vi "Set Controller Configuration.vi"(8 "error in (no error)":errorcluster, 11 "Server Controller in":refnum<class "Server Controller.lvclass">) -> (0 "error out":errorcluster, 3 "Server Controller out":refnum<class "Server Controller.lvclass">)   [LabVIEW 2026, in "Server Controller.lvlib" / "Server Controller.lvclass"]
uses:
  Server Controller.lvclass
  C:/Users/E2013170/Documents/GitHub/Measurement-Utility-Reference/source/framework/Controller/Controller.lvclass
  Server Config.lvclass
  framework/Controller/Controller.lvclass/Controller.ctl
  Server Config.lvclass/Server Config.ctl
  Server Controller.lvclass/Server Controller.ctl
  framework/Controller/Controller.lvclass
  configuration/Configuration.lvclass
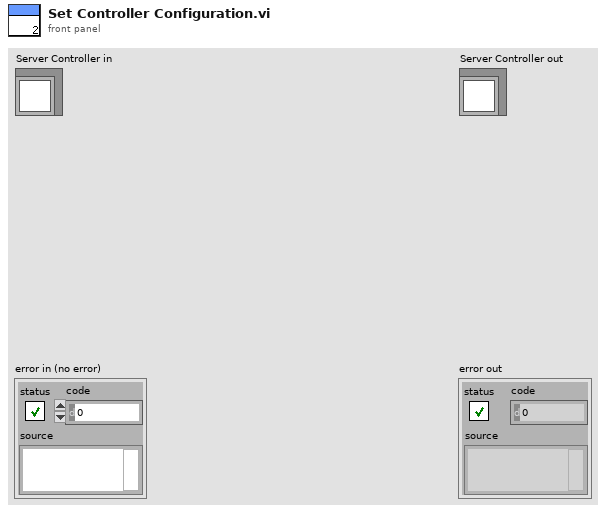
[diagram p1: front panel]
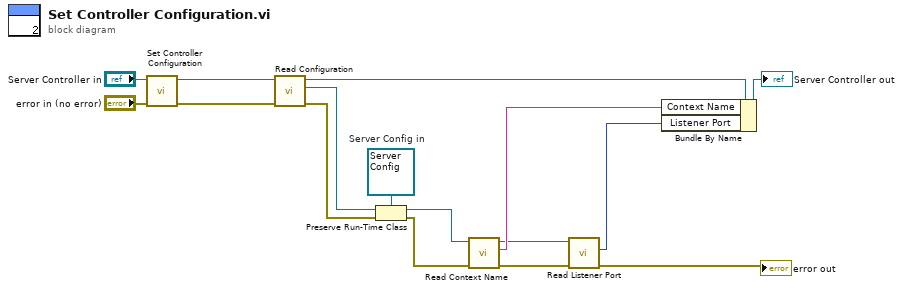
[diagram p0: block diagram]
diagram:
  w12 = refnum<class "Server Config.lvclass"> refnum  # Server Config in
  n1 = call-parent "Set Controller Configuration.vi"("error in (no error)"="error in (no error)", "Controller in"="Server Controller in") -> ("error out"=w14:errorcluster, "Controller out"=w10:refnum<class "Server Controller.lvclass">)  [unwired: 8 in]
  n2 = call "Read Configuration.vi"("error in (no error)"=w14, "Controller in"=w10) -> ("error out"=w2:errorcluster, "Configuration.lvlib:Configuration.lvclass"=w13:refnum<class "Configuration.lvclass">, "Controller out"=w9:refnum<class "Server Controller.lvclass">)  [unwired: 7 in]
  n3 = Preserve Run-Time Class(object in=w13, error in=w2, 2:w12) -> (object out=w11:refnum<class "Server Config.lvclass">, error out=w1:errorcluster)
  n4 = call "Read Context Name.vi"("error in (no error)"=w1, "Server Config in"=w11) -> ("error out"=w4:errorcluster, "Context Name"=w8:string, "Server Config out"=w6:refnum<class "Server Config.lvclass">)  [unwired: 7 in]
  n5 = call "Read Listener Port.vi"("error in (no error)"=w4, "Server Config in"=w6) -> ("error out"=→"error out":errorcluster, "Listener Port"=w5:u16)  [unwired: 7 in, 1 out]
  n6 = Bundle By Name(cluster=w9, "Context Name"=w8, "Listener Port"=w5) -> (→"Server Controller out":refnum<class "Server Controller.lvclass">)
